vi "myRIO v1.0 Build MUX Configuration PWM.vi"(11 "Channel":T4) -> (2 "Configuration Bitmask Array":bool[][](array[boolean]), 3 "Channel Reservation List":T1)   [LabVIEW 2021]
uses:
  <vilib>/myRIO/Common/Instrument Driver Framework/myRIO v1.0/PWM/typedefs/PWM Channels Enum.ctl
  <vilib>/myRIO/Common/Instrument Driver Framework/myRIO v1.0/Resource Manager/typedefs/myRIO v1.0 Channel Reservation List.ctl
  <vilib>/myRIO/Common/Instrument Driver Framework/myRIO v1.0/Resource Manager/typedefs/myRIO v1.0 Channel Reservation Info.ctl
  <vilib>/myRIO/Common/Instrument Driver Framework/myRIO v1.0/Resource Manager/typedefs/myRIO v1.0 Connector List.ctl
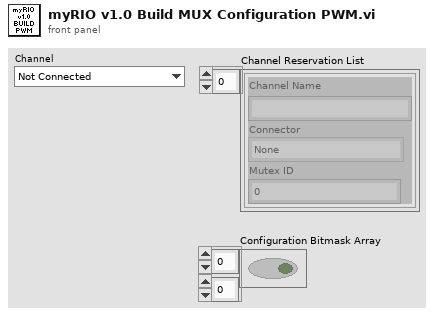
[diagram p1: front panel]
types:
  T1 = typedef "myRIO v1.0 Channel Reservation List.ctl" = T2[]
  T2 = typedef "myRIO v1.0 Channel Reservation Info.ctl" = cluster{"Channel Name":string, "Connector":T3, "Mutex ID":i32}
  T3 = typedef "myRIO v1.0 Connector List.ctl" = enum32{"None", "ConnectorA", "ConnectorB", "ConnectorC"}
  T4 = typedef "PWM Channels Enum.ctl" = enum16{"Not Connected", "C/PWM0", "C/PWM1", "A/PWM0", "A/PWM1", "A/PWM2", "A/PWM3", "A/PWM4", "A/PWM5", "A/PWM6", "A/PWM7", "A/PWM8", "A/PWM9", "A/PWM10", "A/PWM11", "A/PWM12", "A/PWM13", "A/PWM14", "A/PWM15", "A/PWM16", "A/PWM17", "A/PWM18", "A/PWM19", "B/PWM0", "B/PWM1", "B/PWM2", "B/PWM3", "B/PWM4", "B/PWM5", "B/PWM6", "B/PWM7", "B/PWM8", "B/PWM9", "B/PWM10", "B/PWM11", "B/PWM12", "B/PWM13", "B/PWM14", "B/PWM15", "B/PWM16", "B/PWM17", "B/PWM18", "B/PWM19", "PWM/PWM0", "PWM/PWM1", "PWM/PWM2", "PWM/PWM3", "PWM/PWM4", "PWM/PWM5", "PWM/PWM6", "PWM/PWM7", "PWM/PWM8", "PWM/PWM9"}
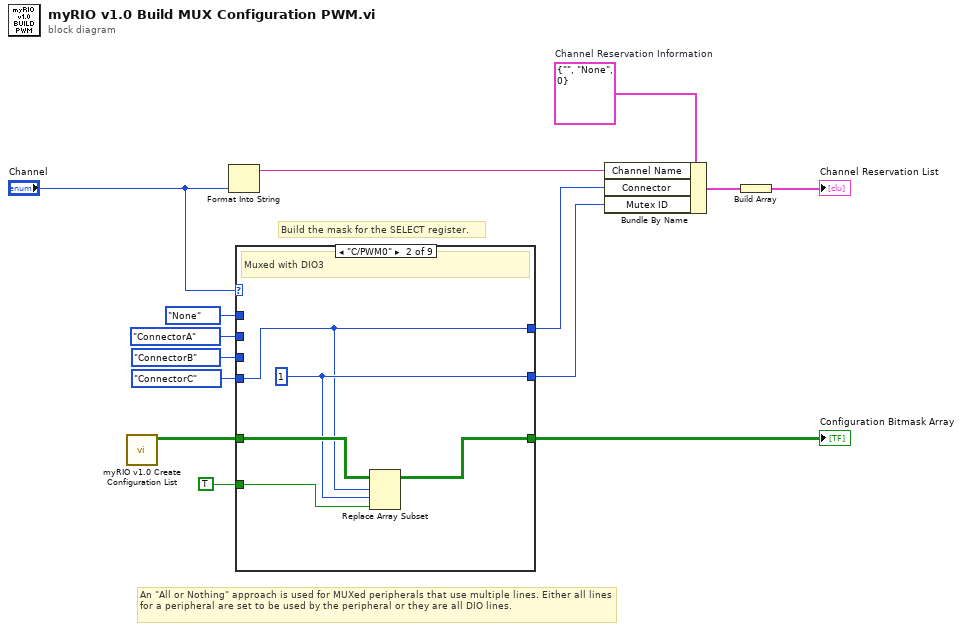
[diagram p0: block diagram]
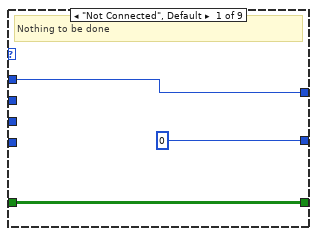
[diagram p2: hidden frame]
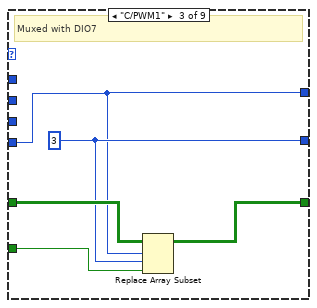
[diagram p3: hidden frame]
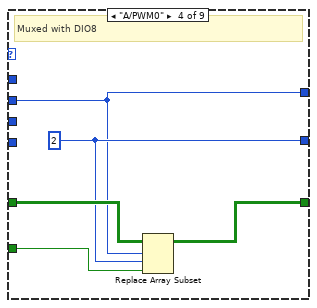
[diagram p4: hidden frame]
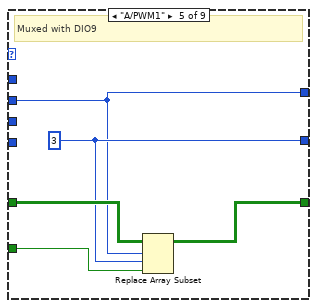
[diagram p5: hidden frame]
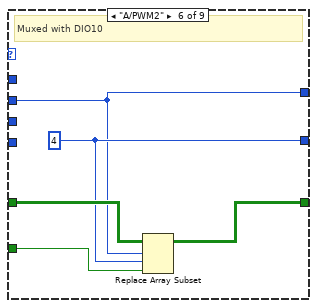
[diagram p6: hidden frame]
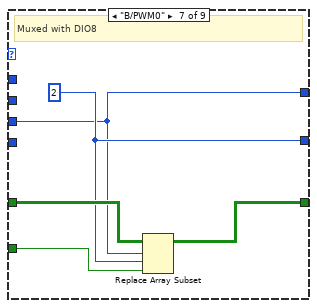
[diagram p7: hidden frame]
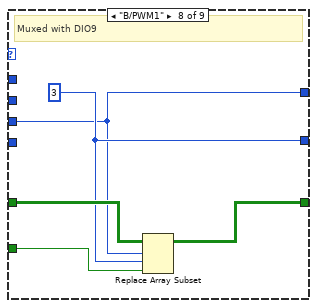
[diagram p8: hidden frame]
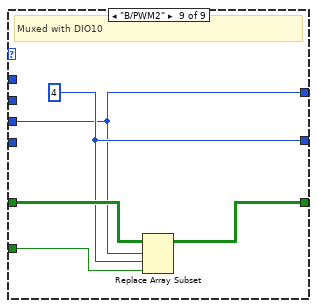
[diagram p9: hidden frame]
diagram:
  w7 = T2 {"Channel Name"="", "Connector"=enum."None", "Mutex ID"=0}  # Channel Reservation Information
  # "An \"All or Nothing\" approach is used for MUXed peripherals that use multiple lines. Either all lines for a peripheral are set to be used by the peripheral or they are all DIO lines."
  # "Build the mask for the SELECT register."
  n1 = call <vilib>:"myRIO v1.0 Create Configuration List.vi"() -> ("Bitmask Array"=w8:bool[][])  [unwired: 11 in]
  n2 = Format Into String("Channel") -> (resulting string=w4:string)  [unwired: 3 in, 1 out]
  n3 = case shown="\"C/PWM0\"" "Channel" {
    tunnel: w8 -> [w17 w22 w27 w32 w37 w42 w47 w52 w57]
    tunnel: [w17 w21 w26 w31 w36 w41 w46 w51 w56] -> w11
    tunnel: myRIO_v1.0_Connector_List."None" ("Connector List") -> [w16 _ _ _ _ _ _ _ _]
    tunnel: myRIO_v1.0_Connector_List."ConnectorA" ("Connector List") -> [_ _ _ w28 w33 w38 _ _ _]
    tunnel: TRUE ("new element/subarray") -> [_ w20 w25 w30 w35 w40 w45 w50 w55]
    tunnel: myRIO_v1.0_Connector_List."ConnectorB" ("Connector List") -> [_ _ _ _ _ _ w43 w48 w53]
    tunnel: myRIO_v1.0_Connector_List."ConnectorC" ("Connector List") -> [_ w18 w23 _ _ _ _ _ _]
    tunnel: [0 ("index") w19 w24 w29 w34 w39 w44 w49 w54] -> w1
    tunnel: [w16 w18 w23 w28 w33 w38 w43 w48 w53] -> w2
    frame "Not Connected", Default {
      # "Nothing to be done"
    }
    frame "C/PWM0" {
      w19 = 1 ("index")
      # "Muxed with DIO3"
      n4 = Replace Array Subset(array=w22, new element=w20, index (row)=w18, index (col)=w19) -> (w21:bool[][])
    }
    frame "C/PWM1" {
      w24 = 3 ("index")
      # "Muxed with DIO7"
      n5 = Replace Array Subset(array=w27, new element=w25, index (row)=w23, index (col)=w24) -> (w26:bool[][])
    }
    frame "A/PWM0" {
      w29 = 2 ("index")
      # "Muxed with DIO8"
      n6 = Replace Array Subset(array=w32, new element=w30, index (row)=w28, index (col)=w29) -> (w31:bool[][])
    }
    frame "A/PWM1" {
      w34 = 3 ("index")
      # "Muxed with DIO9"
      n7 = Replace Array Subset(array=w37, new element=w35, index (row)=w33, index (col)=w34) -> (w36:bool[][])
    }
    frame "A/PWM2" {
      w39 = 4 ("index")
      # "Muxed with DIO10"
      n8 = Replace Array Subset(array=w42, new element=w40, index (row)=w38, index (col)=w39) -> (w41:bool[][])
    }
    frame "B/PWM0" {
      w44 = 2 ("index")
      # "Muxed with DIO8"
      n9 = Replace Array Subset(array=w47, new element=w45, index (row)=w43, index (col)=w44) -> (w46:bool[][])
    }
    frame "B/PWM1" {
      w49 = 3 ("index")
      # "Muxed with DIO9"
      n10 = Replace Array Subset(array=w52, new element=w50, index (row)=w48, index (col)=w49) -> (w51:bool[][])
    }
    frame "B/PWM2" {
      w54 = 4 ("index")
      # "Muxed with DIO10"
      n11 = Replace Array Subset(array=w57, new element=w55, index (row)=w53, index (col)=w54) -> (w56:bool[][])
    }
  }
  "Configuration Bitmask Array" <- w11
  n12 = Bundle By Name(cluster=w7, "Channel Name"=w4, "Connector"=w2, "Mutex ID"=w1) -> (w6:T2)
  n13 = Build Array(w6) -> (→"Channel Reservation List":T2[])
